vi "Scan Engine EtherCAT Generic Slave.vi"(8 "error in (no error)":errorcluster, 11 "Node Ptr":T1 format="%.0x") -> (0 "error out":errorcluster)   [LabVIEW 2016, in "Scan Engine Custom Device.lvlib"]
uses:
  Scan Engine Custom Device.lvlib
  <vilib>/NI Veristand/Custom Device API/Custom Device API.lvlib
  NationalInstruments.VeriStand.SystemDefinitionAPI
  <vilib>/NI Veristand/Custom Device API/Custom Device Item Ref.ctl
panel:
  out "ToString":string
  in  "Export to XML":bool
  in  "Prepend":bool caption="Prepend slave position to name"
  in  "SHDocVw.IWebBrowser2":refnum<k7>(container)
  in  "Slave Position":u16
  in  "Header":cluster{"Section Name":string}={"Section Name"="EtherCAT Slave"}
  in  "Name":string
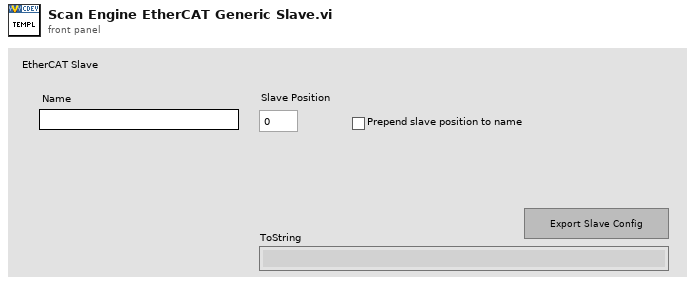
[diagram p1: front panel]
types:
  T1 = typedef "Custom Device API.lvlib/Custom Device Item Ref.ctl" = u64
  T2 = typedef "Custom Device API.lvlib/Custom Device Commands.ctl" = enum16{"Default", "Item renamed", "Shutdown", "Dynamic button pressed"}
  T3 = typedef "Custom Device API.lvlib/Custom Device Pointer.ctl" = refnum<k24>
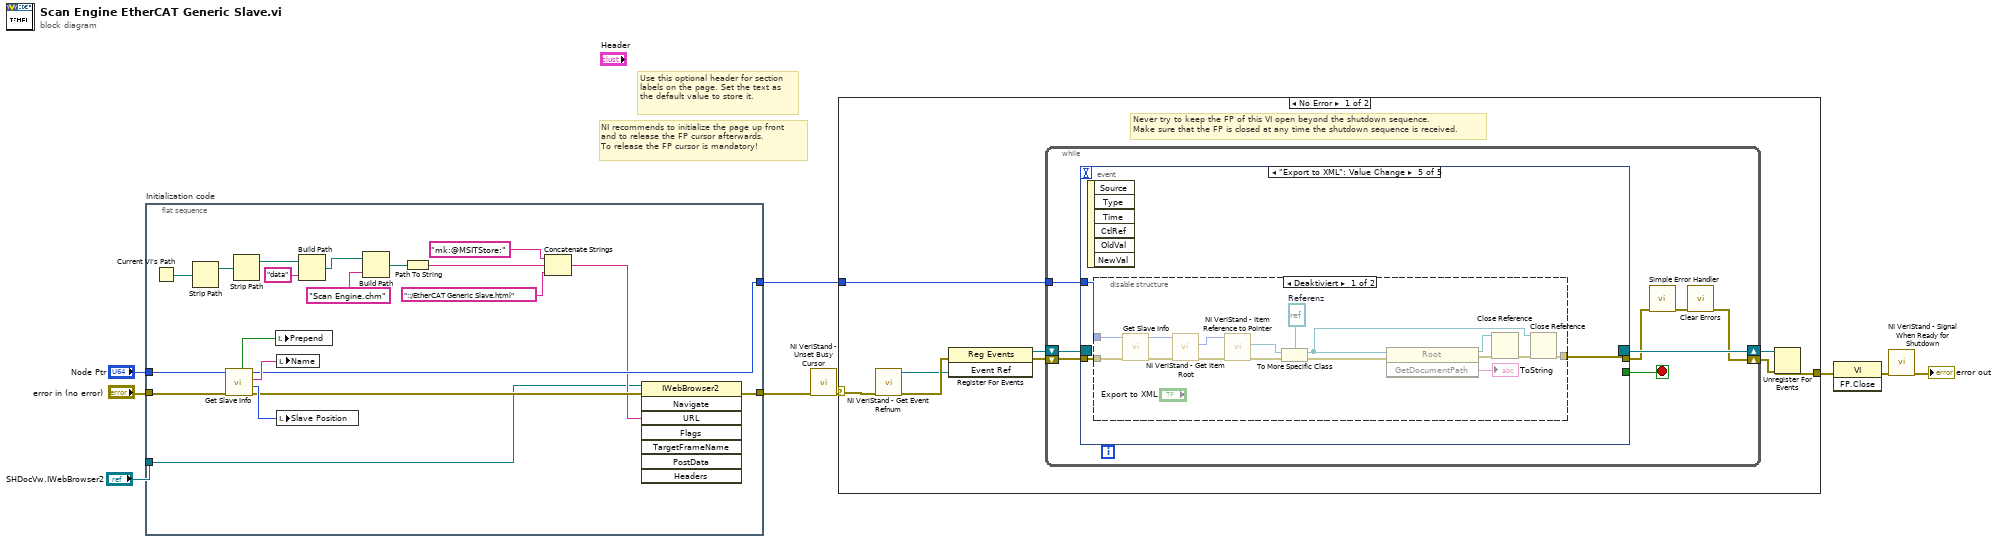
[diagram p0: block diagram]
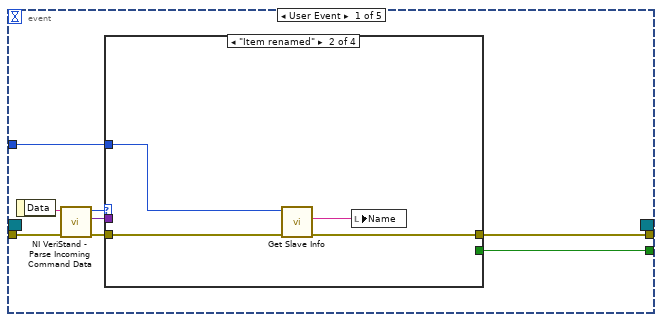
[diagram p2: hidden frame]
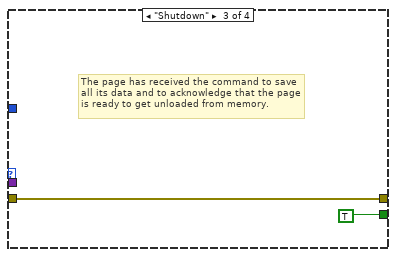
[diagram p4: hidden frame]
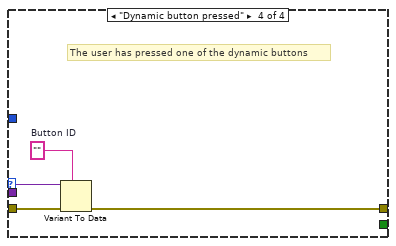
[diagram p5: hidden frame]
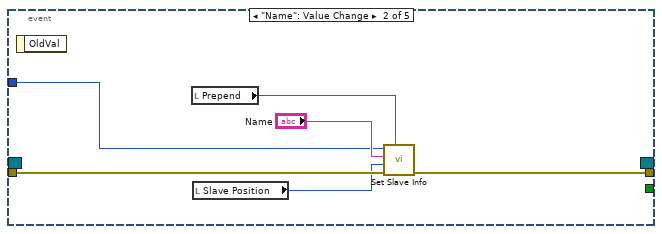
[diagram p6: hidden frame]
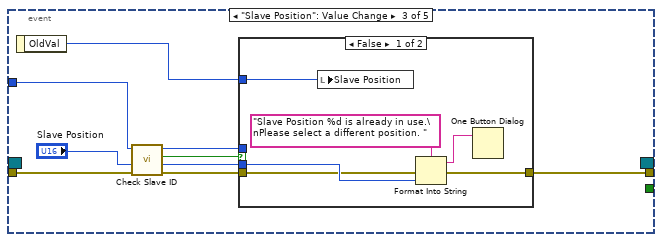
[diagram p7: hidden frame]
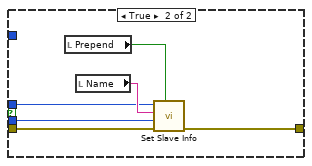
[diagram p8: hidden frame]
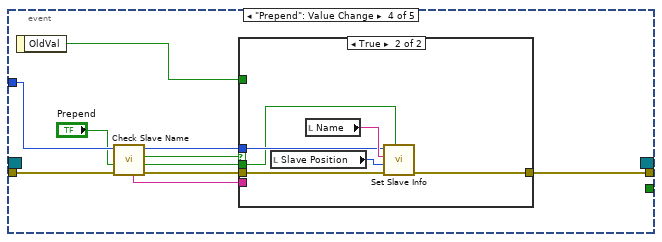
[diagram p9: hidden frame]
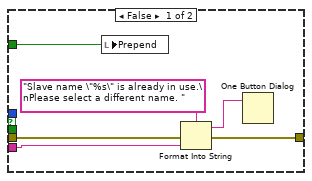
[diagram p10: hidden frame]
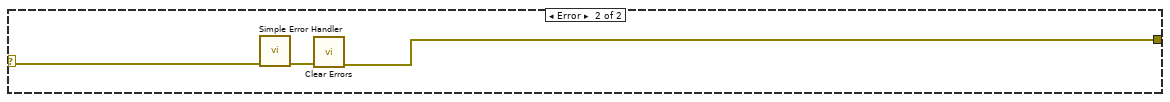
[diagram p12: hidden frame]
diagram:
  # "Use this optional header for section labels on the page. Set the text as the default value to store it."
  # "NI recommends to initialize the page up front\nand to release the FP cursor afterwards.\nTo release the FP cursor is mandatory!"
  n1 = flat-sequence "Initialization code" {
    tunnel: "error in (no error)" -> [w25]
    tunnel: "Node Ptr" -> [w26]
    tunnel: [w13] -> w5
    tunnel: [w27] -> w2
    tunnel: "SHDocVw.IWebBrowser2" -> [w11]
    frame #0 {
      n2 = Current VI's Path() -> (path=w16:path)
      n3 = Strip Path(path=w16) -> (stripped path=w17:path)  [unwired: 1 out]
      n4 = call "Get Slave Info.vi"("error in (no error)"=w25, "Item Ref in"=w26) -> ("error out"=w14:errorcluster, "Slave #"=w28:u16, "Slave Name"=w29:string, "Item Ref out"=w27:T1, "Prepend"=w10:bool)  [unwired: 5 in]
      n5 = Strip Path(path=w17) -> (stripped path=w22:path)  [unwired: 1 out]
      n6 = local write "Prepend"(w10) -> ()
      n7 = local write "Name"(w29) -> ()
      n8 = local write "Slave Position"(w28) -> ()
      n9 = Build Path(base path=w22, name or relative path="data") -> (appended path=w23:path)
      n10 = Build Path(base path=w23, name or relative path="Scan Engine.chm") -> (appended path=w20:path)
      n11 = Path To String(path=w20) -> (string=w19:string)
      n12 = Concatenate Strings("mk:@MSITStore:" ("string"), w19, "::/EtherCAT Generic Slave.html" ("name or relative path")) -> (w12:string)
      n13 = invoke class="IWebBrowser2" method="Navigate"(reference=w11, error in=w14, "URL"=w12) -> (error out=w13:errorcluster)  [unwired: 5 in, 7 out]
    }
  }
  n14 = call <vilib>:"NI VeriStand - Unset Busy Cursor.vi"("error in (no error)"=w5) -> ("error out"=w4:errorcluster)  [unwired: 10 out]
  n15 = case shown="No Error" w4 {
    selector: w4 -> [w30 w136]
    tunnel: [w35 w134] -> w9
    tunnel: w2 -> [w31 _]
    frame No Error {
      # "Never try to keep the FP of this VI open beyond the shutdown sequence.\nMake sure that the FP is closed at any time the shutdown sequence is received."
      n16 = call <vilib>:"NI VeriStand - Get Event Refnum.vi"("error in (no error)"=w30) -> ("error out"=w38:errorcluster, "Event Ref"=w34:refnum<user-event>)  [unwired: 9 out]
      n17 = register-events(error in=w38, w34) -> (reference out=w32:refnum<event-registration>, error out=w33:errorcluster)  [unwired: 1 in]
      n18 = while {
        tunnel: w31 -> [w42]
        shift-right: [w39] -> w36
        shift-left: w33 -> [w45]
        shift-right: [w46] -> w37
        shift-left: w32 -> [w44]
        stop <- w43 stop-if-true
        n19 = event shown="[4] \"Export to XML\": Value Change" {
          selector: w44 -> [_ _ _ _ _]
          dyn-events: [_ _ _ _ _] -> w46
          timeout: _ -> [_ _ _ _ _]
          tunnel: w45 -> [w54 w69 w74 w100 w117]
          tunnel: [w50 _ _ _ _] -> w43
          tunnel: [w49 w70 w72 w101 w115] -> w41
          tunnel: w42 -> [w48 w68 w76 w99 w116]
          event User Event {
            n20 = event-data() -> ("Data"=w53:string)  [unwired: 1 out]
            n21 = call <vilib>:"NI VeriStand - Parse Incoming Command Data.vi"("error in (no error)"=w54, "Incoming data"=w53) -> ("error out"=w52:errorcluster, "Outgoing data"=w47:variant, "Action"=w51:T2)  [unwired: 7 out]
            n22 = case shown="\"Item renamed\"" w51 {
              tunnel: w52 -> [w55 w59 w60 w65]
              tunnel: [_ _ TRUE _] -> w50
              tunnel: [w55 w58 w60 w62] -> w49
              tunnel: w48 -> [_ w56 _ _]
              tunnel: w47 -> [_ _ _ w64]
              frame "Default", Default {
              }
              frame "Item renamed" {
                n23 = call "Get Slave Info.vi"("error in (no error)"=w59, "Item Ref in"=w56) -> ("error out"=w58:errorcluster, "Slave Name"=w57:string)  [unwired: 5 in, 3 out]
                n24 = local write "Name"(w57) -> ()
              }
              frame "Shutdown" {
                # "The page has received the command to save all its data and to acknowledge that the page is ready to get unloaded from memory."
              }
              frame "Dynamic button pressed" {
                w63 = ""  # Button ID
                # "The user has pressed one of the dynamic buttons"
                n25 = Variant To Data(error in=w65, type=w63, Variant=w64) -> (error out=w62:errorcluster)  [unwired: 1 out]
              }
            }
          }
          event "Name": Value Change {
            n26 = event-data() -> ()  [unwired: 2 out]
            n27 = local read "Prepend"() -> (w66:bool)
            n28 = local read "Slave Position"() -> (w67:u16)
            n29 = call "Set Slave Info.vi"("Prepend"=w66, "error in (no error)"=w69, "Slave #"=w67, "Slave Name"="Name", "Item Ref in"=w68) -> ("error out"=w70:errorcluster)  [unwired: 5 in, 1 out]
          }
          event "Slave Position": Value Change {
            n30 = event-data() -> ("OldVal"=w73:u16)  [unwired: 1 out]
            n31 = call "Check Slave ID.vi"("error in (no error)"=w74, "Slave ID in"="Slave Position", "Item Ref in"=w76) -> ("error out"=w80:errorcluster, "Slave ID out"=w78:u16, "Available?"=w79:bool, "Item Ref out"=w77:T1)  [unwired: 5 in]
            n32 = case shown="False" w79 {
              tunnel: [w82 w92] -> w72
              tunnel: w80 -> [w83 w91]
              tunnel: w77 -> [_ w88]
              tunnel: w78 -> [w85 w90]
              tunnel: w73 -> [w81 _]
              frame False {
                n33 = local write "Slave Position"(w81) -> ()
                n34 = Format Into String(format string="Slave Position %d is already in use.\nPlease select a different position. ", error in=w83, w85) -> (resulting string=w84:string, error out=w82:errorcluster)  [unwired: 1 in]
                n35 = One Button Dialog(message=w84) -> ()  [unwired: 1 in, 1 out]
              }
              frame True {
                n36 = local read "Prepend"() -> (w87:bool)
                n37 = local read "Name"() -> (w89:string)
                n38 = call "Set Slave Info.vi"("Prepend"=w87, "error in (no error)"=w91, "Slave #"=w90, "Slave Name"=w89, "Item Ref in"=w88) -> ("error out"=w92:errorcluster)  [unwired: 5 in, 1 out]
              }
            }
          }
          event "Prepend": Value Change {
            n39 = event-data() -> ("OldVal"=w102:bool)  [unwired: 1 out]
            n40 = call "Check Slave Name.vi"("error in (no error)"=w100, "Prepend in"="Prepend", "Item Ref in"=w99) -> ("error out"=w95:errorcluster, "Prepend out"=w94:bool, "Available?"=w96:bool, "Item Ref out"=w97:T1, "Slave Name"=w93:string)  [unwired: 4 in]
            n41 = case shown="True" w96 {
              tunnel: [w105 w114] -> w101
              tunnel: w95 -> [w106 w113]
              tunnel: w97 -> [_ w111]
              tunnel: w94 -> [_ w110]
              tunnel: w102 -> [w108 _]
              tunnel: w93 -> [w103 _]
              frame False {
                n42 = local write "Prepend"(w108) -> ()
                n43 = Format Into String(format string="Slave name \"%s\" is already in use.\nPlease select a different name. ", error in=w106, w103) -> (resulting string=w104:string, error out=w105:errorcluster)  [unwired: 1 in]
                n44 = One Button Dialog(message=w104) -> ()  [unwired: 1 in, 1 out]
              }
              frame True {
                n45 = local read "Slave Position"() -> (w109:u16)
                n46 = local read "Name"() -> (w112:string)
                n47 = call "Set Slave Info.vi"("Prepend"=w110, "error in (no error)"=w113, "Slave #"=w109, "Slave Name"=w112, "Item Ref in"=w111) -> ("error out"=w114:errorcluster)  [unwired: 5 in, 1 out]
              }
            }
          }
          event "Export to XML": Value Change {
            n48 = event-data() -> ()  [unwired: 7 out]
            n49 = disable-structure shown="Deaktiviert" {
              disable-tunnel: w117 -> [w133 _]
              disable-tunnel: w116 -> [w132 _]
              disable-tunnel: [w127 _] -> w115
              frame Disabled {
                w121 = refnum<k24> refnum  # Referenz
                n50 = call "Get Slave Info.vi"("error in (no error)"=w133, "Item Ref in"=w132) -> ("error out"=w131:errorcluster, "Item Ref out"=w123:T1)  [unwired: 5 in, 3 out]
                n51 = call <vilib>:"NI VeriStand - Get Item Root.vi"("error in (no error)"=w131, "Item Ref in"=w123) -> ("error out"=w124:errorcluster, "Root Ref out"=w120:T1)  [unwired: 6 in, 2 out]
                n52 = call <vilib>:"NI VeriStand - Item Reference to Pointer.vi"("error in (no error)"=w124, "Item Ref in"=w120) -> ("error out"=w126:errorcluster, "Node Pointer"=w119:T3)  [unwired: 6 in, 2 out]
                n53 = To More Specific Class(target class=w121, reference=w119, error in=w126) -> (specific class reference=w122:refnum<k24>, error out=w125:errorcluster)
                n54 = invoke class="Root" method="GetDocumentPath"(reference=w122, error in=w125) -> (reference out=w129:refnum<k24>, error out=w130:errorcluster, "GetDocumentPath"=→"ToString":string)  [unwired: 1 in]
                n55 = Close Reference(reference=w129, error in (no error)=w130) -> (error out=w128:errorcluster)
                n56 = Close Reference(reference=w122, error in (no error)=w128) -> (error out=w127:errorcluster)
              }
              frame Enabled {
              }
            }
          }
        }
        n57 = call <vilib>:"Simple Error Handler.vi"("error in (no error)"=w41) -> ("error out"=w40:errorcluster)  [unwired: 1 in, 7 out]
        n58 = call <vilib>:"Clear Errors.vi"("error in (no error)"=w40) -> ("error out"=w39:errorcluster)  [unwired: 1 in, 5 out]
      }
      n59 = Unregister For Events(event registration refnum=w37, error in=w36) -> (error out=w35:errorcluster)
    }
    frame Error {
      n60 = call <vilib>:"Simple Error Handler.vi"("error in (no error)"=w136) -> ("error out"=w135:errorcluster)  [unwired: 1 in, 7 out]
      n61 = call <vilib>:"Clear Errors.vi"("error in (no error)"=w135) -> ("error out"=w134:errorcluster)  [unwired: 1 in, 5 out]
    }
  }
  n62 = invoke class="VI" method="FP.Close"(error in=w9) -> (error out=w8:errorcluster)  [unwired: 2 in, 2 out]
  n63 = call <vilib>:"NI VeriStand - Signal When Ready for Shutdown.vi"("error in (no error)"=w8) -> ("error out"=→"error out":errorcluster)  [unwired: 10 out]
